vi "CPT Bootprozess 12.1.vi"(9 "FifoNo":u16=1, 11 "Boot File Relative Referenz":string) -> (1 "Starte Prozess - error out":errorcluster, 3 "Device No. out":u16 format="%.0x")   [LabVIEW 2015]
panel:
  out "Fir":errorcluster
  in  "Device No.":u16=336 format="%.0x"
  out "Lade Prozess":errorcluster
  out "Free Memory - error out":errorcluster
  out "Free Memory [byte]":i32
  out "Workload - error out":errorcluster
  out "Workload":i16
  out "Processor type (1011 = T11)":u16
  out "Prozessor Typ":errorcluster
  out "Bootprozess":errorcluster
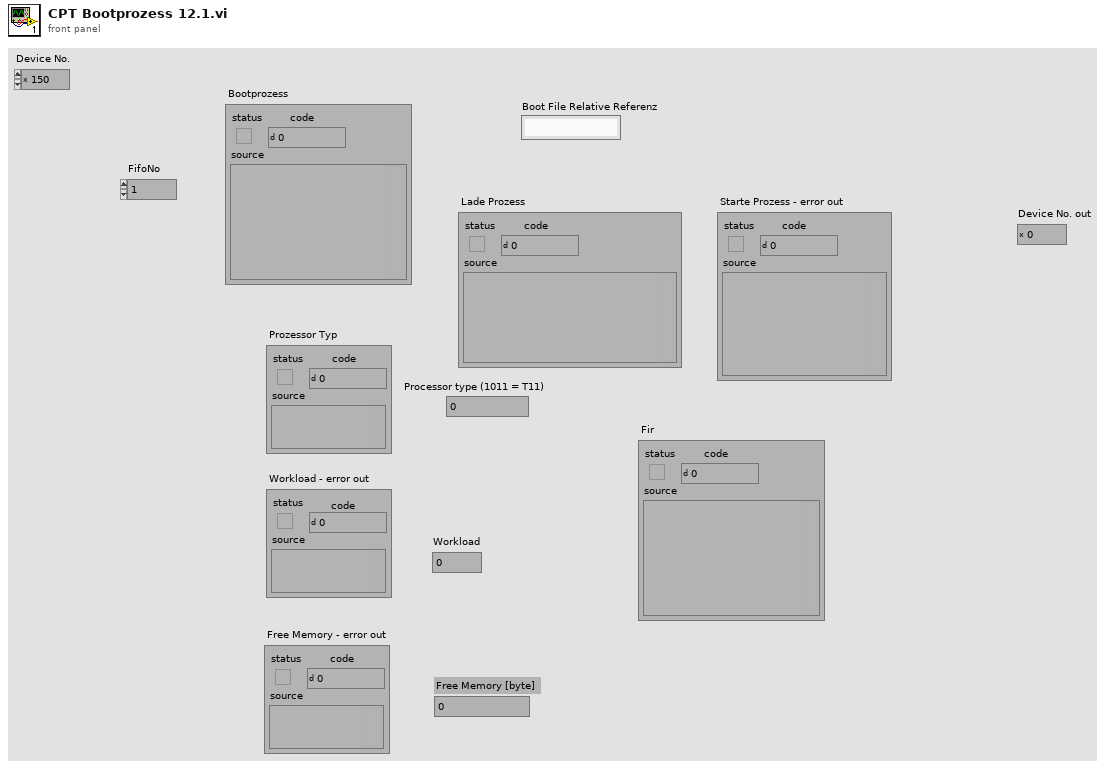
[diagram p1: front panel]
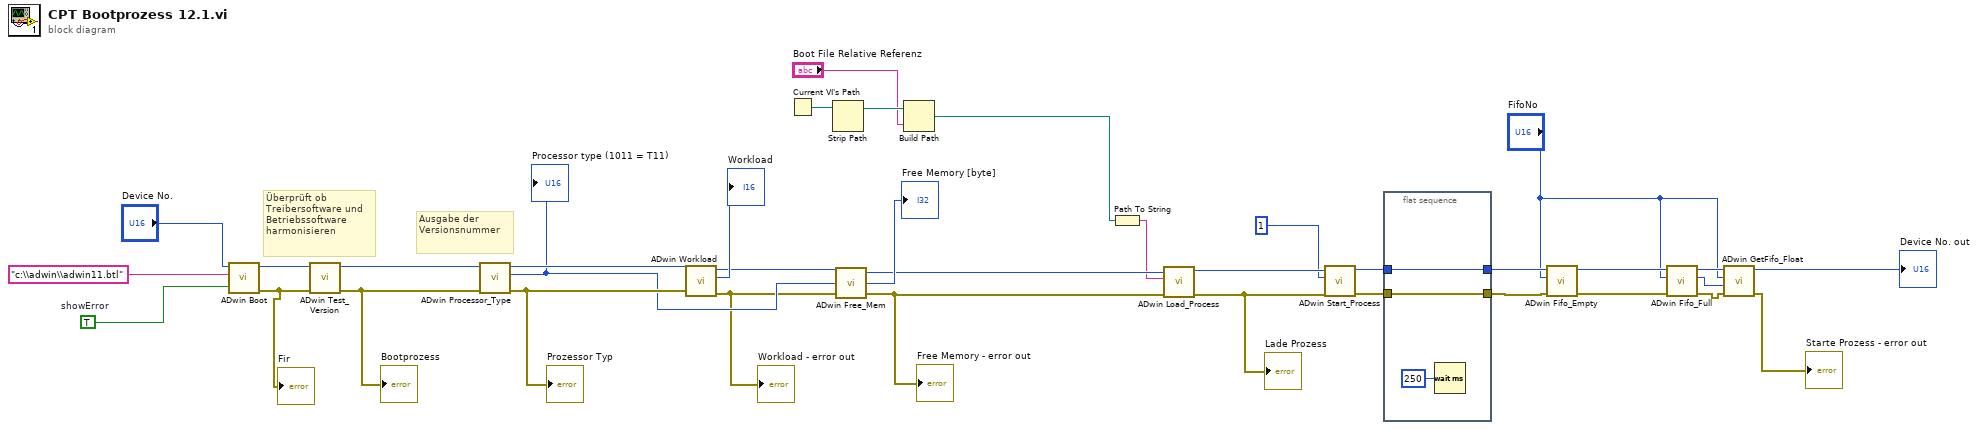
[diagram p0: block diagram]
diagram:
  w35 = TRUE  # showError
  # "Ausgabe der Versionsnummer"
  # "Überprüft ob Treibersoftware und Betriebssoftware harmonisieren"
  n1 = call "ADwin Boot.vi"("showError"=w35, "Filename"="c:\\adwin\\adwin11.btl", "Device No."="Device No.") -> ("error out"=w6:errorcluster, "Device No. out"=w34:u16)  [unwired: 6 in, 1 out]
  "Fir" <- w6
  n2 = call "ADwin Test_Version.vi"("error in (no error)"=w6, "Device No."=w34) -> ("error out"=w33:errorcluster, "Device No. out"=w32:u16)  [unwired: 7 in, 1 out]
  "Bootprozess" <- w33
  n3 = call "ADwin Processor_Type.vi"("error in (no error)"=w33, "Device No."=w32) -> ("error out"=w29:errorcluster, "Processor type"=w27:u16, "Device No. out"=w31:u16)  [unwired: 7 in]
  "Prozessor Typ" <- w29
  "Processor type (1011 = T11)" <- w27
  n4 = call "ADwin Workload.vi"("error in (no error)"=w29, "Device No."=w31) -> ("error out"=w26:errorcluster, "Workload"=→"Workload":i16, "Device No. out"=w28:u16)  [unwired: 7 in]
  "Workload - error out" <- w26
  n5 = Current VI's Path() -> (path=w5:path)
  n6 = Strip Path(path=w5) -> (stripped path=w4:path)  [unwired: 1 out]
  n7 = call "ADwin Free_Mem.vi"("error in (no error)"=w26, "Processor"=w27, "Device No."=w28) -> ("error out"=w23:errorcluster, "Memory"=→"Free Memory [byte]":i32, "Device No. out"=w24:u16)
  "Free Memory - error out" <- w23
  n8 = Build Path(base path=w4, name or relative path="Boot File Relative Referenz") -> (appended path=w2:path)
  n9 = Path To String(path=w2) -> (string=w1:string)
  n10 = call "ADwin Load_Process.vi"("error in (no error)"=w23, "Filename"=w1, "Device No."=w24) -> ("error out"=w21:errorcluster, "Device No. out"=w22:u16)  [unwired: 6 in, 1 out]
  "Lade Prozess" <- w21
  n11 = call "ADwin Start_Process.vi"("error in (no error)"=w21, "ProcessNumber"=1, "Device No."=w22) -> ("error out"=w16:errorcluster, "Device No. out"=w17:u16)  [unwired: 6 in, 1 out]
  n12 = flat-sequence {
    tunnel: [w38] -> w15
    tunnel: w17 -> [w38]
    tunnel: [w37] -> w14
    tunnel: w16 -> [w37]
    frame #0 {
      n13 = Wait (ms)(milliseconds to wait=u32 250) -> ()  [unwired: 1 out]
    }
  }
  n14 = call "ADwin Fifo_Empty.vi"("error in (no error)"=w14, "FifoNo"="FifoNo", "Device No."=w15) -> ("error out"=w12:errorcluster, "Device No. out"=w13:u16)  [unwired: 2 in, 1 out]
  n15 = call "ADwin Fifo_Full.vi"("error in (no error)"=w12, "FifoNo"="FifoNo", "Device No."=w13) -> ("error out"=w8:errorcluster, "Count"=w18:i32, "Device No. out"=w19:u16)  [unwired: 6 in]
  n16 = call "ADwin GetFifo_Float.vi"("error in (no error)"=w8, "count"=w18, "FifoNo"="FifoNo", "Device No."=w19) -> ("error out"=→"Starte Prozess - error out":errorcluster, "Device No. out"=→"Device No. out":u16)  [unwired: 4 in, 2 out]
